vi "Arduino_Hygrometer_configure.vi"() -> ()   [LabVIEW 2020]
uses:
  Instrument drivers/Arduino/ctls_and_globals/Arduino tx msg cluster.ctl
panel:
  out "Output":string
  in  "P_offset (mb) [0.1 .... 25.5]*":sgl=9.5
  in  "Sampling rate (Hz)":u16(ring)=1 items=["10", "1", "0.1", "0.01"]
  out "Status comment":string
  in  "Port":refnum<visa-resource-name>="COM18"
  in  "Address":u8=17
  # "Use this vi to configure the Hygrometer\nThis value is retained in EEPROM and recalled on power-up."
  # "* The Enflo Lab is around 60m above sea level. It is therefore necessary to subtract\n7.2mb from any sea level meteorological value. The offset here should be adjusted\nto match the altitude-adjusted sea level pressure information."
  # "PN 23/09/2014"
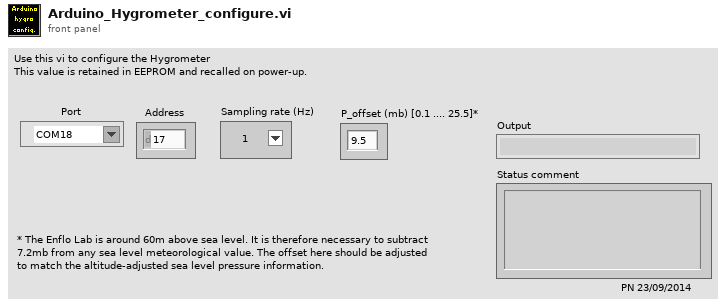
[diagram p1: front panel]
types:
  T1 = typedef "Arduino tx msg cluster.ctl" = cluster{"dest":u8, "A/D/C/I":string, "R/W":string, "chan":u8, "val (float)":sgl}
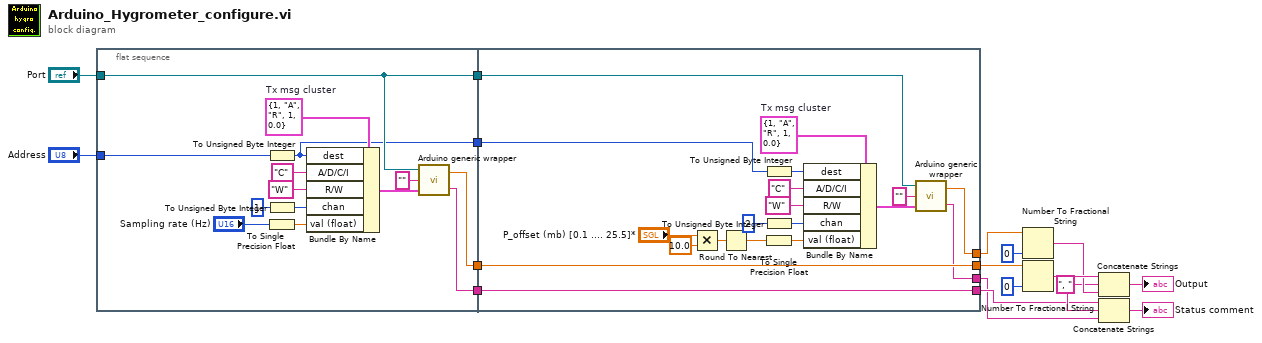
[diagram p0: block diagram]
diagram:
  w7 = ", "
  n1 = flat-sequence {
    tunnel: "Address" -> [w23]
    tunnel: "Port" -> [w24]
    tunnel: [w24] -> w15
    tunnel: [w22] -> w14
    tunnel: [w21] -> w13
    tunnel: [w20] -> w12
    tunnel: w15 -> [w43]
    tunnel: w14 -> [w42]
    tunnel: w13 -> [w35]
    tunnel: w12 -> [w36]
    tunnel: [w36] -> w11
    tunnel: [w35] -> w6
    tunnel: [w34] -> w5
    tunnel: [w33] -> w10
    frame #0 {
      w30 = T1 {"dest"=1, "A/D/C/I"="A", "R/W"="R", "chan"=1, "val (float)"=0.0}  # Tx msg cluster
      n2 = To Unsigned Byte Integer(number=w23) -> (unsigned 8bit integer=w22:u8)
      n3 = To Unsigned Byte Integer(number=u8 1) -> (unsigned 8bit integer=w25:u8)
      n4 = To Single Precision Float(number="Sampling rate (Hz)") -> (single precision float=w27:sgl)
      n5 = Bundle By Name(cluster=w30, "dest"=w22, "A/D/C/I"="C" ("A/D"), "R/W"="W", "chan"=w25, "val (float)"=w27) -> (w26:T1)
      n6 = call "Arduino generic wrapper.vi"("Tx msg cluster"=w26, "Channel Name"="", "Port name"=w24) -> ("Scan comment"=w21:string, "Output"=w20:dbl)
    }
    frame #1 {
      w50 = T1 {"dest"=1, "A/D/C/I"="A", "R/W"="R", "chan"=1, "val (float)"=0.0}  # Tx msg cluster
      n7 = Multiply(x="P_offset (mb) [0.1 .... 25.5]*", y=sgl 10.0) -> (x*y=w38:sgl)
      n8 = Round To Nearest(number=w38) -> (nearest integer value=w37:sgl)
      n9 = To Unsigned Byte Integer(number=w42) -> (unsigned 8bit integer=w48:u8)
      n10 = To Unsigned Byte Integer(number=u8 2) -> (unsigned 8bit integer=w49:u8)
      n11 = To Single Precision Float(number=w37) -> (single precision float=w46:sgl)
      n12 = Bundle By Name(cluster=w50, "dest"=w48, "A/D/C/I"="C" ("A/D"), "R/W"="W", "chan"=w49, "val (float)"=w46) -> (w47:T1)
      n13 = call "Arduino generic wrapper.vi"("Tx msg cluster"=w47, "Channel Name"="", "Port name"=w43) -> ("Scan comment"=w34:string, "Output"=w33:dbl)
    }
  }
  n14 = Number To Fractional String(number=w10, precision (6)=i16 0) -> (F-format string=w8:string)  [unwired: 2 in]
  n15 = Number To Fractional String(number=w11, precision (6)=i16 0) -> (F-format string=w9:string)  [unwired: 2 in]
  n16 = Concatenate Strings(w9, w7, w8) -> (→"Output":string)
  n17 = Concatenate Strings(w6, w7, w5) -> (→"Status comment":string)
